vi "Set Producer Values.vi"(8 "error in":errorcluster, 9 "Producer Ch":T2[](array[typedef])=[{"Error.STS"=0, "OutputEnable.STS"=0, "ControlMode.STS"=0, "Temperature.AV"=0.0, "Pressure.AV"=0.0, "Flow.AV"=0.0}], 10 "Producer Control":T1, 11 "Chiller Cluster.lvclass in":refnum<class "Chiller Cluster.lvclass">) -> (0 "error out":errorcluster, 3 "Chiller Cluster.lvclass out":refnum<class "Chiller Cluster.lvclass">)   [LabVIEW 2023, in "Chiller Cluster.lvclass"]
uses:
  Chiller Cluster.lvclass
  Producer Ch.ctl
  Producer Control.ctl
  Chiller Cluster.lvclass/Chiller Cluster.ctl
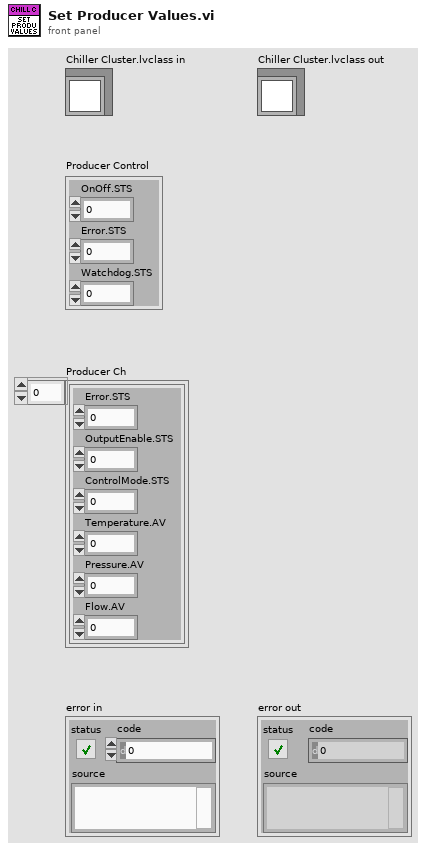
[diagram p1: front panel]
types:
  T1 = typedef "Chiller Cluster.lvclass/Producer Control.ctl" = cluster{"OnOff.STS":i32, "Error.STS":i32, "Watchdog.STS":i32}
  T2 = typedef "Chiller Cluster.lvclass/Producer Ch.ctl" = cluster{"Error.STS":i32, "OutputEnable.STS":i32, "ControlMode.STS":u16, "Temperature.AV":dbl, "Pressure.AV":dbl, "Flow.AV":dbl}
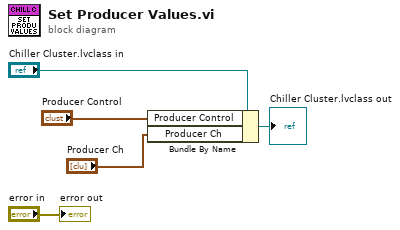
[diagram p0: block diagram]
diagram:
  n1 = Bundle By Name(cluster="Chiller Cluster.lvclass in", "Producer Control"="Producer Control", "Producer Ch"="Producer Ch") -> (→"Chiller Cluster.lvclass out":refnum<class "Chiller Cluster.lvclass">)
  "error out" <- "error in"
